vi "counter_sum.vi"(8 "error in":errorcluster) -> (0 "error IO":errorcluster, 1 "Number of Hours":dbl, 2 "Third Detector Sum":i64, 3 "First Detector Sum":i64)   [LabVIEW 2013]
uses:
  <vilib>/addons/database/_DB Variant To Data/Database Variant To Data.xnode
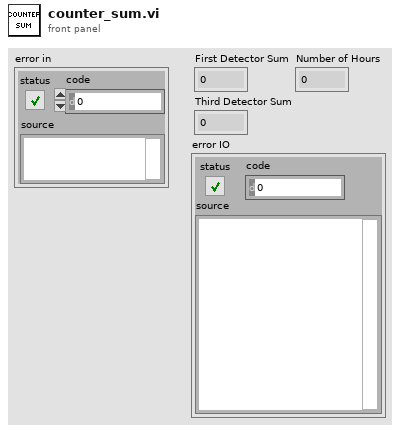
[diagram p1: front panel]
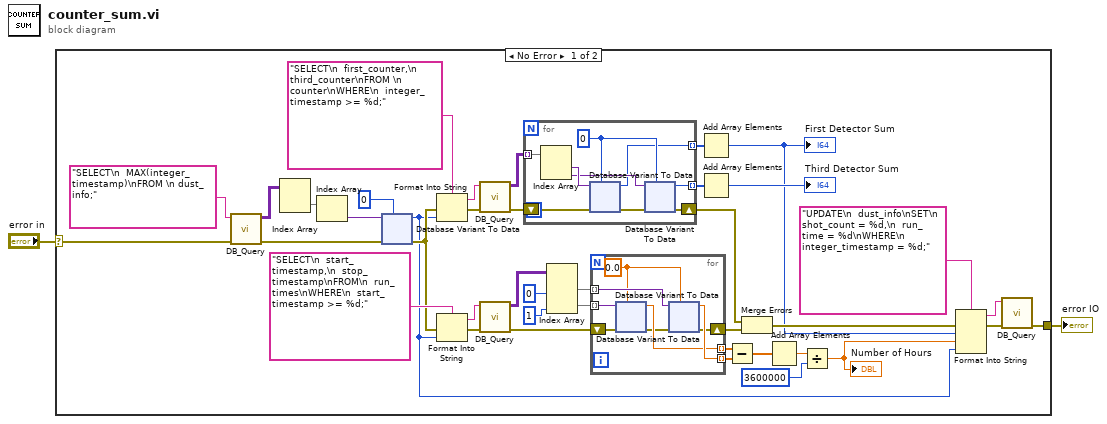
[diagram p0: block diagram]
diagram:
  n1 = case shown="No Error" "error in" {
    selector: "error in" -> [w25 w220]
    tunnel: [w27 w220] -> w1
    frame No Error {
      n2 = call "DB_Query.vi"("error in (no error)"=w25, "Parameterized Query"="SELECT\n  MAX(integer_timestamp)\nFROM \n dust_info;" ("SQL query")) -> ("error out"=w21:errorcluster, "Results"=w24:variant[][])  [unwired: 7 in, 1 out]
      n3 = Index Array(array=w24) -> (element=w23:variant[])  [unwired: 2 in]
      n4 = Index Array(array=w23) -> (element=w22:variant)  [unwired: 1 in]
      n5 = xnode "Database Variant To Data"("database variant"=w22, "error in (no error)"=w21, "type"=i64 0) -> ("data"=w3:i64, "error out"=w8:errorcluster)
      n6 = Format Into String(format string="SELECT\n  first_counter,\n  third_counter\nFROM \n counter\nWHERE\n  integer_timestamp >= %d;" ("SQL query"), error in=w8, w3) -> (resulting string=w18:string, error out=w12:errorcluster)  [unwired: 1 in]
      n7 = Format Into String(format string="SELECT\n  start_timestamp,\n  stop_timestamp\nFROM\n  run_times\nWHERE\n  start_timestamp >= %d;" ("SQL query"), error in=w8, w3) -> (resulting string=w9:string, error out=w7:errorcluster)  [unwired: 1 in]
      n8 = call "DB_Query.vi"("error in (no error)"=w12, "Parameterized Query"=w18) -> ("error out"=w11:errorcluster, "Results"=w17:variant[][])  [unwired: 7 in, 1 out]
      n9 = call "DB_Query.vi"("error in (no error)"=w7, "Parameterized Query"=w9) -> ("error out"=w6:errorcluster, "Results"=w5:variant[][])  [unwired: 7 in, 1 out]
      n10 = for {
        tunnel: w17 -> [w123] mode=indexing
        shift-right: [w119] -> w10
        shift-left: w11 -> [w121]
        tunnel: [w116] -> w15 mode=indexing
        tunnel: [w115] -> w16 mode=indexing
        w122 = i64 0
        n11 = Index Array(array=w123) -> (element #1=w118:variant, element #2=w117:variant)  [unwired: 2 in]
        n12 = xnode "Database Variant To Data"("database variant"=w118, "error in (no error)"=w121, "type"=w122) -> ("data"=w115:i64, "error out"=w120:errorcluster)
        n13 = xnode "Database Variant To Data"("database variant"=w117, "error in (no error)"=w120, "type"=w122) -> ("data"=w116:i64, "error out"=w119:errorcluster)
      }
      n14 = Index Array(array=w5, index (col) #1=0 ("disabled index (col)"), index (col) #2=1 ("index (col)")) -> (element #1=w38:variant[], element #2=w39:variant[])  [unwired: 2 in]
      n15 = for {
        tunnel: w38 -> [w50] mode=indexing
        tunnel: w39 -> [w49] mode=indexing
        tunnel: [w46] -> w33 mode=indexing
        tunnel: [w48] -> w34 mode=indexing
        shift-right: [w43] -> w4
        shift-left: w6 -> [w47]
        w45 = 0.0
        n16 = xnode "Database Variant To Data"("database variant"=w49, "error in (no error)"=w47, "type"=w45) -> ("data"=w46:dbl, "error out"=w44:errorcluster)
        n17 = xnode "Database Variant To Data"("database variant"=w50, "error in (no error)"=w44, "type"=w45) -> ("data"=w48:dbl, "error out"=w43:errorcluster)
      }
      n18 = Add Array Elements(numeric array=w16) -> (sum=w13:i64)
      "First Detector Sum" <- w13
      n19 = Add Array Elements(numeric array=w15) -> (sum=→"Third Detector Sum":i64)
      n20 = Subtract(x=w33, y=w34) -> (x-y=w37:dbl[])
      n21 = Merge Errors(w10, w4) -> (w28:errorcluster)
      n22 = Add Array Elements(numeric array=w37) -> (sum=w36:dbl)
      n23 = Divide(x=w36, y=i64 3600000) -> (x/y=w26:dbl)
      "Number of Hours" <- w26
      n24 = Format Into String(format string="UPDATE\n  dust_info\nSET\n  shot_count = %d,\n  run_time = %d\nWHERE\n  integer_timestamp = %d;" ("Parameterized Query"), error in=w28, w13, w26, w3) -> (resulting string=w30:string, error out=w31:errorcluster)  [unwired: 1 in]
      n25 = call "DB_Query.vi"("error in (no error)"=w31, "Parameterized Query"=w30) -> ("error out"=w27:errorcluster)  [unwired: 7 in, 2 out]
    }
    frame Error {
    }
  }
  "error IO" <- w1
